vi "ENPH354_A3Q2_20213140.vi"() -> ()   [LabVIEW 2020]
panel:
  out "Total number of letters":dbl
  out "Letter Frequency Values":cluster{"String":string, "Numeric":dbl}[](array[cluster])
  out "Waveform Graph":dbl[](graph)
  in  "file path (use dialog)":path
  in  "stop":bool
  # "Author: Jose Ramon Gonzalez (20213140)\nENPH354 Assignment 3 Q2"
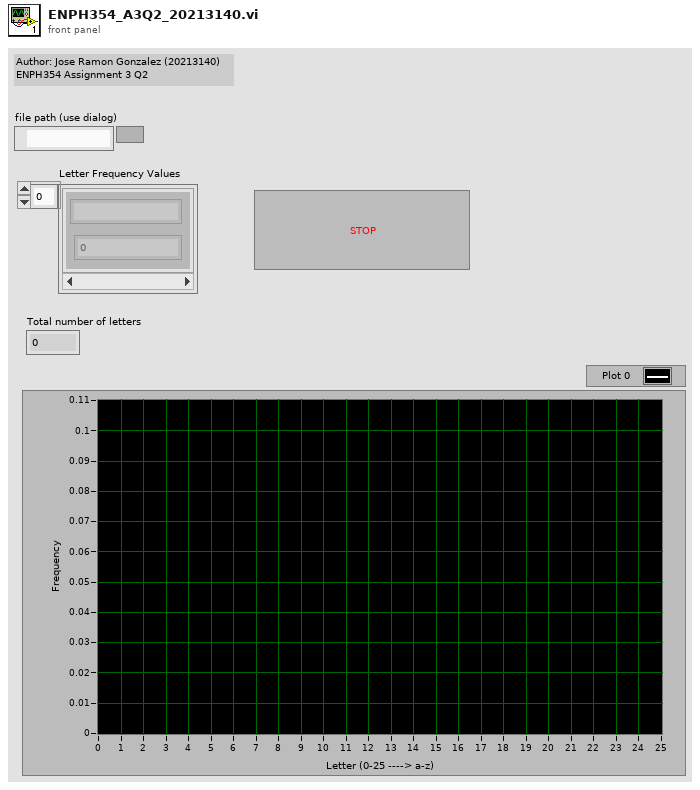
[diagram p1: front panel]
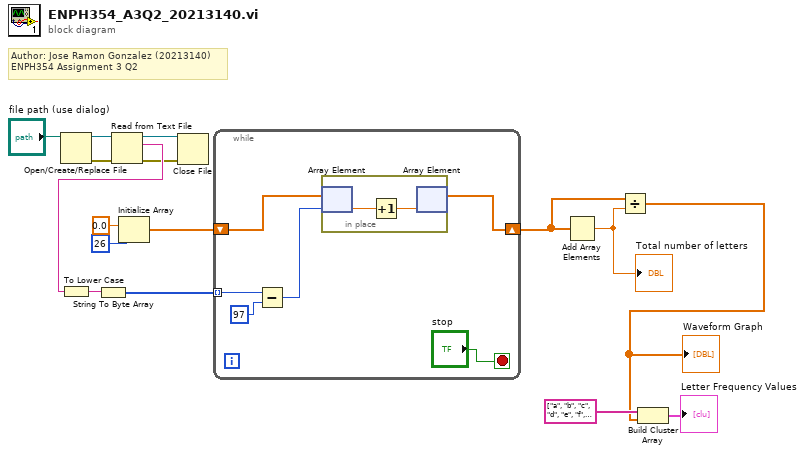
[diagram p0: block diagram]
diagram:
  # "Author: Jose Ramon Gonzalez (20213140)\nENPH354 Assignment 3 Q2"
  n1 = Open/Create/Replace File(file path (use dialog)="file path (use dialog)") -> (refnum out=w14:refnum<file>, error out=w2:errorcluster)  [unwired: 5 in, 1 out]
  n2 = Read from Text File(file (use dialog)=w14, error in=w2) -> (refnum out=w15:refnum<file>, text=w13:string, error out=w1:errorcluster)  [unwired: 2 in, 1 out]
  n3 = To Lower Case(string=w13) -> (all lower case string=w12:string)
  n4 = String To Byte Array(string=w12) -> (unsigned byte array=w11:u8[])
  n5 = Initialize Array(0.0 ("element"), 26 ("dimension size")) -> (w8:dbl[])
  n6 = Close File(refnum=w15, error in=w1) -> ()  [unwired: 2 out]
  n7 = while {
    tunnel: w11 -> [w22] mode=indexing
    shift-right: [w17] -> w7
    shift-left: w8 -> [w19]
    stop <- "stop" stop-if-true
    n8 = Subtract(x=w22, y=u8 97) -> (x-y=w18:u8)
    n9 = in-place {
      n10 = in-place-array #1(w19, w18) -> (w24:dbl)
      n11 = Increment(x=w24) -> (x+1=w23:dbl)
      n12 = in-place-array #1(w23) -> (w17:dbl[])  [unwired: 1 out]
    }
  }
  n13 = Add Array Elements(numeric array=w7) -> (sum=w4:dbl)
  "Total number of letters" <- w4
  n14 = Divide(x=w7, y=w4) -> (x/y=w3:dbl[])
  "Waveform Graph" <- w3
  n15 = Build Cluster Array(string[] ["a", "b", "c", "d", "e", "f", "g", "h", "i", "j", "k", "l", "m", "n", "o", "p", "q", "r", "s", "t", "u", "v", "w", "x", "y", "z"] ("array"), w3) -> (→"Letter Frequency Values":cluster{"string":string, "element":dbl}[])
